vi "XPS_DelayLine_Initialize.vi"(11 "Group Name":string="Group2") -> (2 "XPS Error":errorcluster, 3 "XPS Reference":refnum<k24>)   [LabVIEW 2025]
uses:
  C:/Users/user/Nutstore/1/Nutstore/fs-TA/Library/Newport.XPS.CommandInterface.dll
  Library/Newport.XPS.CommandInterface.dll
panel:
  out "ms":u32
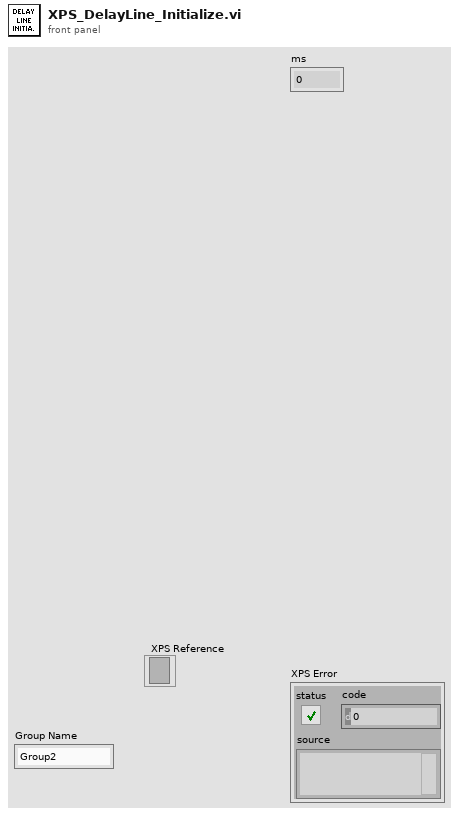
[diagram p1: front panel]
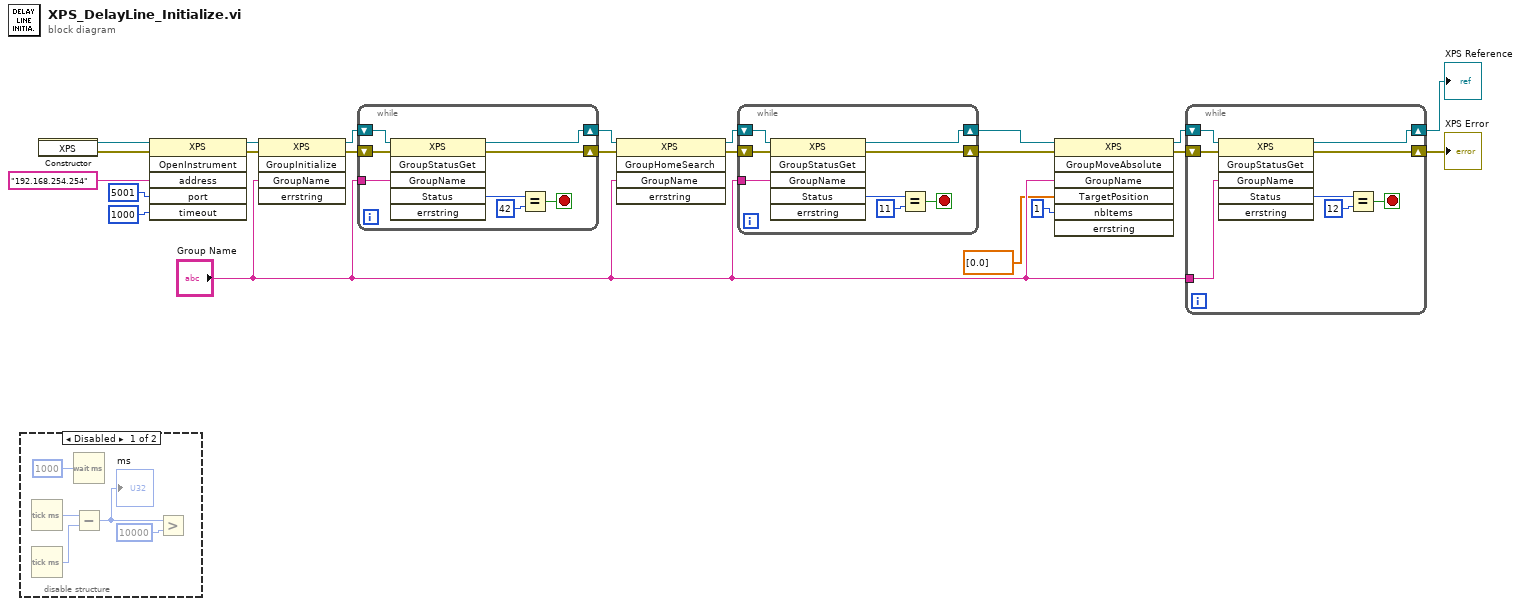
[diagram p0: block diagram]
diagram:
  n1 = disable-structure shown="Disabled" {
    frame Disabled {
      n2 = Tick Count (ms)() -> (millisecond timer value=w27:u32)
      n3 = Tick Count (ms)() -> (millisecond timer value=w23:u32)
      n4 = Wait (ms)(milliseconds to wait=u32 1000) -> ()  [unwired: 1 out]
      n5 = Subtract(x=w27, y=w23) -> (x-y=w26:u32)
      "ms" <- w26
      n6 = Greater?(x=w26, y=u32 10000) -> ()  [unwired: 1 out]
    }
    frame Enabled {
    }
  }
  n7 = constructor class="XPS"() -> (reference out=w22:refnum<k24>, error out=w21:errorcluster)  [unwired: 3 in, 1 out]
  n8 = invoke class="XPS" method="OpenInstrument"(reference=w22, error in=w21, "address"="192.168.254.254", "port"=5001, "timeout"=1000) -> (reference out=w20:refnum<k24>, error out=w19:errorcluster)  [unwired: 1 in, 4 out]
  n9 = invoke class="XPS" method="GroupInitialize"(reference=w20, error in=w19, "GroupName"="Group Name") -> (reference out=w15:refnum<k24>, error out=w11:errorcluster)  [unwired: 2 in, 3 out]
  n10 = while {
    tunnel: "Group Name" -> [w31]
    shift-right: [w34] -> w14
    shift-left: w15 -> [w35]
    shift-right: [w32] -> w10
    shift-left: w11 -> [w33]
    stop <- w30 stop-if-true
    n11 = invoke class="XPS" method="GroupStatusGet"(reference=w35, error in=w33, "GroupName"=w31) -> (reference out=w34:refnum<k24>, error out=w32:errorcluster, "Status"=w29:i32)  [unwired: 3 in, 3 out]
    n12 = Equal?(x=w29, y=42) -> (x = y?=w30:bool)
  }
  n13 = invoke class="XPS" method="GroupHomeSearch"(reference=w14, error in=w10, "GroupName"="Group Name") -> (reference out=w13:refnum<k24>, error out=w9:errorcluster)  [unwired: 2 in, 3 out]
  n14 = while {
    tunnel: "Group Name" -> [w39]
    shift-right: [w42] -> w12
    shift-left: w13 -> [w43]
    shift-right: [w40] -> w8
    shift-left: w9 -> [w41]
    stop <- w36 stop-if-true
    n15 = invoke class="XPS" method="GroupStatusGet"(reference=w43, error in=w41, "GroupName"=w39) -> (reference out=w42:refnum<k24>, error out=w40:errorcluster, "Status"=w37:i32)  [unwired: 3 in, 3 out]
    n16 = Equal?(x=w37, y=11) -> (x = y?=w36:bool)
  }
  n17 = invoke class="XPS" method="GroupMoveAbsolute"(reference=w12, error in=w8, "GroupName"="Group Name", "TargetPosition"=dbl[] [0.0], "nbItems"=1) -> (reference out=w4:refnum<k24>, error out=w3:errorcluster)  [unwired: 2 in, 5 out]
  n18 = while {
    tunnel: "Group Name" -> [w51]
    shift-right: [w47] -> w2
    shift-left: w4 -> [w48]
    shift-right: [w45] -> w1
    shift-left: w3 -> [w46]
    stop <- w44 stop-if-true
    n19 = invoke class="XPS" method="GroupStatusGet"(reference=w48, error in=w46, "GroupName"=w51) -> (reference out=w47:refnum<k24>, error out=w45:errorcluster, "Status"=w49:i32)  [unwired: 3 in, 3 out]
    n20 = Equal?(x=w49, y=12) -> (x = y?=w44:bool)
  }
  "XPS Error" <- w1
  "XPS Reference" <- w2
